vi "Initialize.vi"(8 "error in (no error)":errorcluster, 9 "Reset (True)":bool=TRUE, 10 "ID Query (True)":bool=TRUE, 11 "VISA resource name":refnum<visa-resource-name>) -> (0 "error out":errorcluster, 3 "VISA resource name out":refnum<visa-resource-name>)   [LabVIEW 2012, in "Tektronix DPO MSO 2000 4000 Series.lvlib"]
doc: "Establishes communication with an oscilloscope. This VI optionally performs an instrument identification query and/or resets the oscilloscope. The Initialize VI also configures the oscilloscope to a default state that other instrument driver operations require.\nRun this VI before running other instrument driver VIs for the oscilloscope. You generally need to call the Initialize VI only once, at the beginning of an application."
uses:
  <instrlib>/Tektronix DPO MSO 2000 4000 Series/Tektronix DPO MSO 2000 4000 Series.lvlib
panel:
  # "(C) 2006 - 2013. National Instruments Corporation. ALL RIGHTS RESERVED."
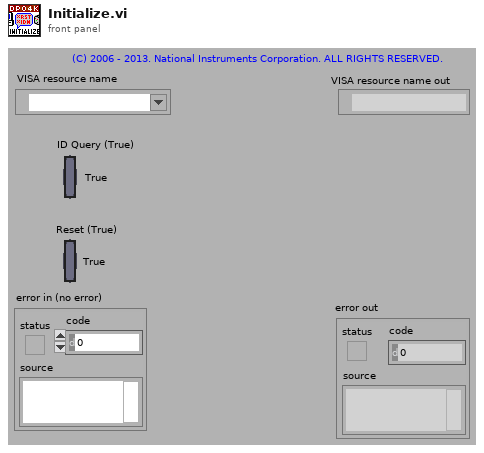
[diagram p1: front panel]
types:
  T1 = enum16{"DPO4104", "DPO4054", "DPO4034", "DPO4032"}
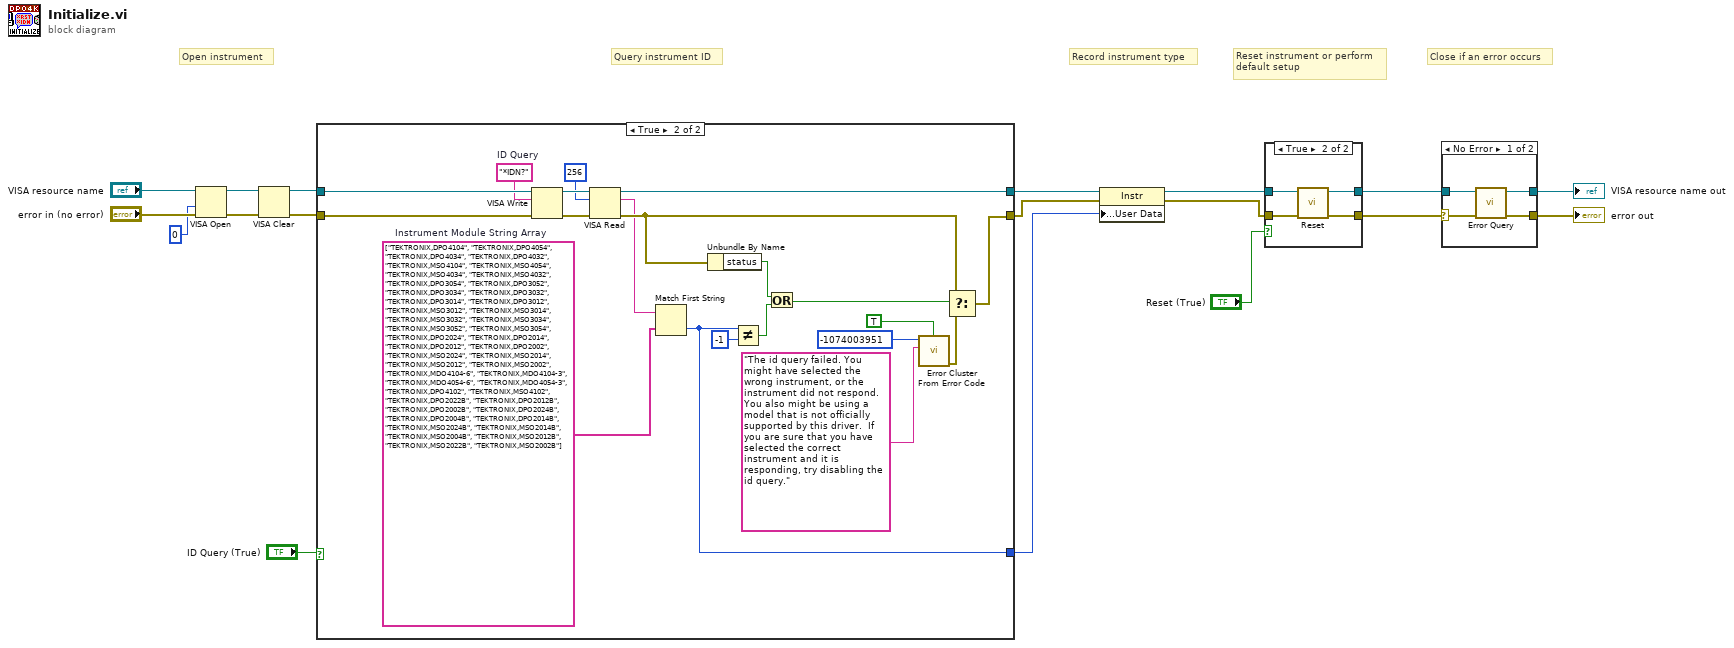
[diagram p0: block diagram]
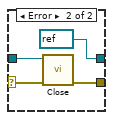
[diagram p2: hidden frame]
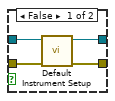
[diagram p3: hidden frame]
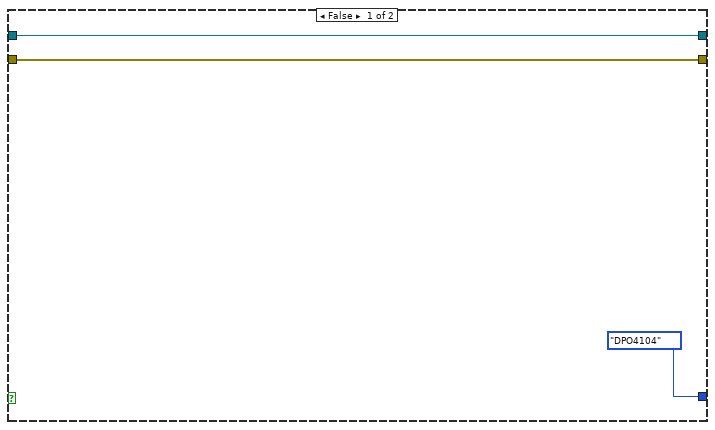
[diagram p4: hidden frame]
diagram:
  # "Record instrument type"
  # "Close if an error occurs"
  # "Query instrument ID"
  # "Reset instrument or perform\ndefault setup"
  # "Open instrument"
  n1 = VISA Open(access mode=u32 0, error in (no error)="error in (no error)", VISA resource name="VISA resource name") -> (VISA resource name=w14:refnum<visa-resource-name>, error out=w13:errorcluster)  [unwired: 2 in]
  n2 = VISA Clear(VISA resource name=w14, error in (no error)=w13) -> (VISA resource name out=w8:refnum<visa-resource-name>, error out=w7:errorcluster)
  n3 = case shown="True" "ID Query (True)" {
    tunnel: [w20 w41] -> w4
    tunnel: [w21 w38] -> w5
    tunnel: w8 -> [w21 w39]
    tunnel: w7 -> [w20 w40]
    tunnel: [T1."DPO4104" ("Instrument Module") w23] -> w1
    frame False {
    }
    frame True {
      w22 = string[] ["TEKTRONIX,DPO4104", "TEKTRONIX,DPO4054", "TEKTRONIX,DPO4034", "TEKTRONIX,DPO4032", "TEKTRONIX,MSO4104", "TEKTRONIX,MSO4054", "TEKTRONIX,MSO4034", "TEKTRONIX,MSO4032", "TEKTRONIX,DPO3054", "TEKTRONIX,DPO3052", "TEKTRONIX,DPO3034", "TEKTRONIX,DPO3032", "TEKTRONIX,DPO3014", "TEKTRONIX,DPO3012", "TEKTRONIX,MSO3012", "TEKTRONIX,MSO3014", "TEKTRONIX,MSO3032", "TEKTRONIX,MSO3034", "TEKTRONIX,MSO3052", "TEKTRONIX,MSO3054", "TEKTRONIX,DPO2024", "TEKTRONIX,DPO2014", "TEKTRONIX,DPO2012", "TEKTRONIX,DPO2002", "TEKTRONIX,MSO2024", "TEKTRONIX,MSO2014", "TEKTRONIX,MSO2012", "TEKTRONIX,MSO2002", "TEKTRONIX,MDO4104-6", "TEKTRONIX,MDO4104-3", "TEKTRONIX,MDO4054-6", "TEKTRONIX,MDO4054-3", "TEKTRONIX,DPO4102", "TEKTRONIX,MSO4102", "TEKTRONIX,DPO2022B", "TEKTRONIX,DPO2012B", "TEKTRONIX,DPO2002B", "TEKTRONIX,DPO2024B", "TEKTRONIX,DPO2004B", "TEKTRONIX,DPO2014B", "TEKTRONIX,MSO2024B", "TEKTRONIX,MSO2014B", "TEKTRONIX,MSO2004B", "TEKTRONIX,MSO2012B", "TEKTRONIX,MSO2022B", "TEKTRONIX,MSO2002B"]  # Instrument Module String Array
      w34 = "*IDN?"  # ID Query
      n4 = VISA Write(VISA resource name=w39, write buffer=w34, error in (no error)=w40) -> (VISA resource name out=w37:refnum<visa-resource-name>, error out=w36:errorcluster)  [unwired: 1 out]
      n5 = VISA Read(VISA resource name=w37, byte count=u32 256, error in (no error)=w36) -> (VISA resource name out=w38:refnum<visa-resource-name>, read buffer=w28:string, error out=w29:errorcluster)  [unwired: 1 out]
      n6 = Match First String(2:w22, 3:w28) -> (0:w23:i32)  [unwired: 1 out]
      n7 = Unbundle By Name(w29) -> ("status"=w26:bool)
      n8 = Not Equal?(x=w23, y=-1) -> (x != y?=w25:bool)
      n9 = Or(x=w26, y=w25) -> (x .or. y?=w24:bool)
      n10 = call <vilib>:"Error Cluster From Error Code.vi"("show call chain? (False)"=TRUE, "error message (\"\")"="The id query failed. You might have selected the wrong instrument, or the instrument did not respond.  You also might be using a model that is not officially supported by this driver.  If you are sure that you have selected the correct instrument and it is responding, try disabling the id query." ("Source (VI Name)"), "error code (0)"=-1074003951 ("Code")) -> ("error out"=w33:errorcluster)  [unwired: 6 in]
      n11 = Select(t=w29, s=w24, f=w33) -> (s? t:f=w41:errorcluster)
    }
  }
  n12 = property class="Instr"(reference=w5, error in=w4, "General Settings:User Data"=w1) -> (reference out=w3:refnum<visa-resource-name>, error out=w2:errorcluster)
  n13 = case shown="True" "Reset (True)" {
    tunnel: w2 -> [w44 w46]
    tunnel: [w43 w49] -> w9
    tunnel: w3 -> [w45 w47]
    tunnel: [w42 w48] -> w10
    frame False {
      n14 = call <instrlib>:"Default Instrument Setup.vi"("error in (no error)"=w44, "VISA resource name"=w45) -> ("error out"=w43:errorcluster, "VISA resource name out"=w42:refnum<visa-resource-name>)  [unwired: 8 in]
    }
    frame True {
      n15 = call <instrlib>:"Reset.vi"("error in (no error)"=w46, "VISA resource name"=w47) -> ("error out"=w49:errorcluster, "VISA resource name out"=w48:refnum<visa-resource-name>)  [unwired: 8 in]
    }
  }
  n16 = case shown="No Error" w9 {
    selector: w9 -> [w51 w55]
    tunnel: w10 -> [w50 w56]
    tunnel: [w53 refnum<visa-resource-name> refnum ("VISA resource name out")] -> w12
    tunnel: [w52 w57] -> w11
    frame No Error {
      n17 = call <instrlib>:"Error Query.vi"("error in (no error)"=w51, "VISA resource name"=w50) -> ("error out"=w52:errorcluster, "VISA resource name out"=w53:refnum<visa-resource-name>)  [unwired: 6 in, 2 out]
    }
    frame Error {
      n18 = call <instrlib>:"Close.vi"("error in (no error)"=w55, "VISA resource name"=w56) -> ("error out"=w57:errorcluster)  [unwired: 9 in]
    }
  }
  "VISA resource name out" <- w12
  "error out" <- w11
